vi "Polaris print label from powered unit.vi"(8 "error in (no error)":errorcluster, 10 "Baud":dbl=115200.0, 11 "VISA Refnum in":refnum<visa-resource-name>="COM11") -> (0 "error out":errorcluster)   [LabVIEW 2013]
panel:
  in  "Check label IMEI to unit?":bool
  out "IP":string
  out "Print Label OK?":bool=TRUE
  in  "Serial Number":u32
  in  "Printer name":string="\\\\LT-85LKFW2\\ZT230-300"
  out "ZPL final":string
  in  "ZPL template":string="\u0010CT~~CD,~CC^~CT~\n^XA~TA000~JSN^LT0^MNW^MTT^PON^PMN^LH0,0^JMA^PR4,4~SD28^JUS^LRN^CI0^XZ\n^FX Start of label zpl^FS\n^XA\n^MMT\n^PW750\n^LL0540\n^LS0\n^FT29,327^A0N,25,24^FH\\^FDNL PN: 1003071^FS\n^FT28,357^A0N,25,24^FH\\^FDIMEI: ImeiImeiImeiIme^FS\n^FT29,388^A0N,25,24^FH\\^FDICCID: EsimEsimEsimEsimEsim^FS\n^FT27,420^A0N,25,24^FH\\^FDSerial: WORKORDER^FS\n^FT28,451^A0N,22,22^FH\\^FDContains FCCID: RI7LE910CXWWX^FS\n^FT27,481^A0N,22,22^FH\\^FDContains IC: 5131A-LE910CXWWX^FS\n^FT359,327^A0N,21,21^FH\\^FDThis device complies with Part 15 of the^FS\n^FT359,353^A0N,21,21^FH\\^FDFCC Rules. Operation is subject to the^FS\n^FT359,379^A0N,21,21^FH\\^FDfollowing two conditions: (1) this device^FS\n^FT359,405^A0N,21,21^FH\\^FDmay not cause harmful interference, and^FS\n^FT359,431^A0N,21,21^FH\\^FD(2) this device must accept any interference^FS\n^FT359,457^A0N,21,21^FH\\^FDreceived, including interference that may^FS\n^FT359,483^A0N,21,21^FH\\^FDcause undesired operation.^FS\n^BY133,132^FT92,195^BXN,6,200,22,22,1,_\n^FH\\^FD4081093        EsimEsimEsimEsimEsim^FS\n^FT117,225^A0N,25,24^FH\\^FD4081093^FS\n^BY133,132^FT482,195^BXN,6,200,22,22,1,_\n^FH\\^FD3286910        ImeiImeiImeiIme^FS\n^FT500,228^A0N,25,24^FH\\^FD3286910^FS\n^FT459,256^A0N,25,24^FH\\^FDImeiImeiImeiIme^FS\n^FT59,253^A0N,25,24^FH\\^FDEsimEsimEsimEsimEsim^FS\n^PQ1,0,1,Y^XZ"
  out "imei":string
  out "eSim ICCID":string
  # "printer1=\\\\\\\\SkywireTestPC1\\ZDesigner ZT230-300dpi ZPL (Copy 1)\nprinter2=\\\\\\\\PucTestPC2\\ZDesigner ZT230-300dpi ZPL\nprinter3=\\\\\\\\NIMBELNKTESTPC3\\ZDesigner GX430t\nprinter4=\\\\\\\\dt-hkn77p2\\ZDesigner ZT230-200dpi ZPL\nprinter5=\\\\\\\\nimbelink-08\\ZDesigner ZT230-300dpi ZPL\nprinter6=\\\\\\\\LT-85LKFW2\\\\"
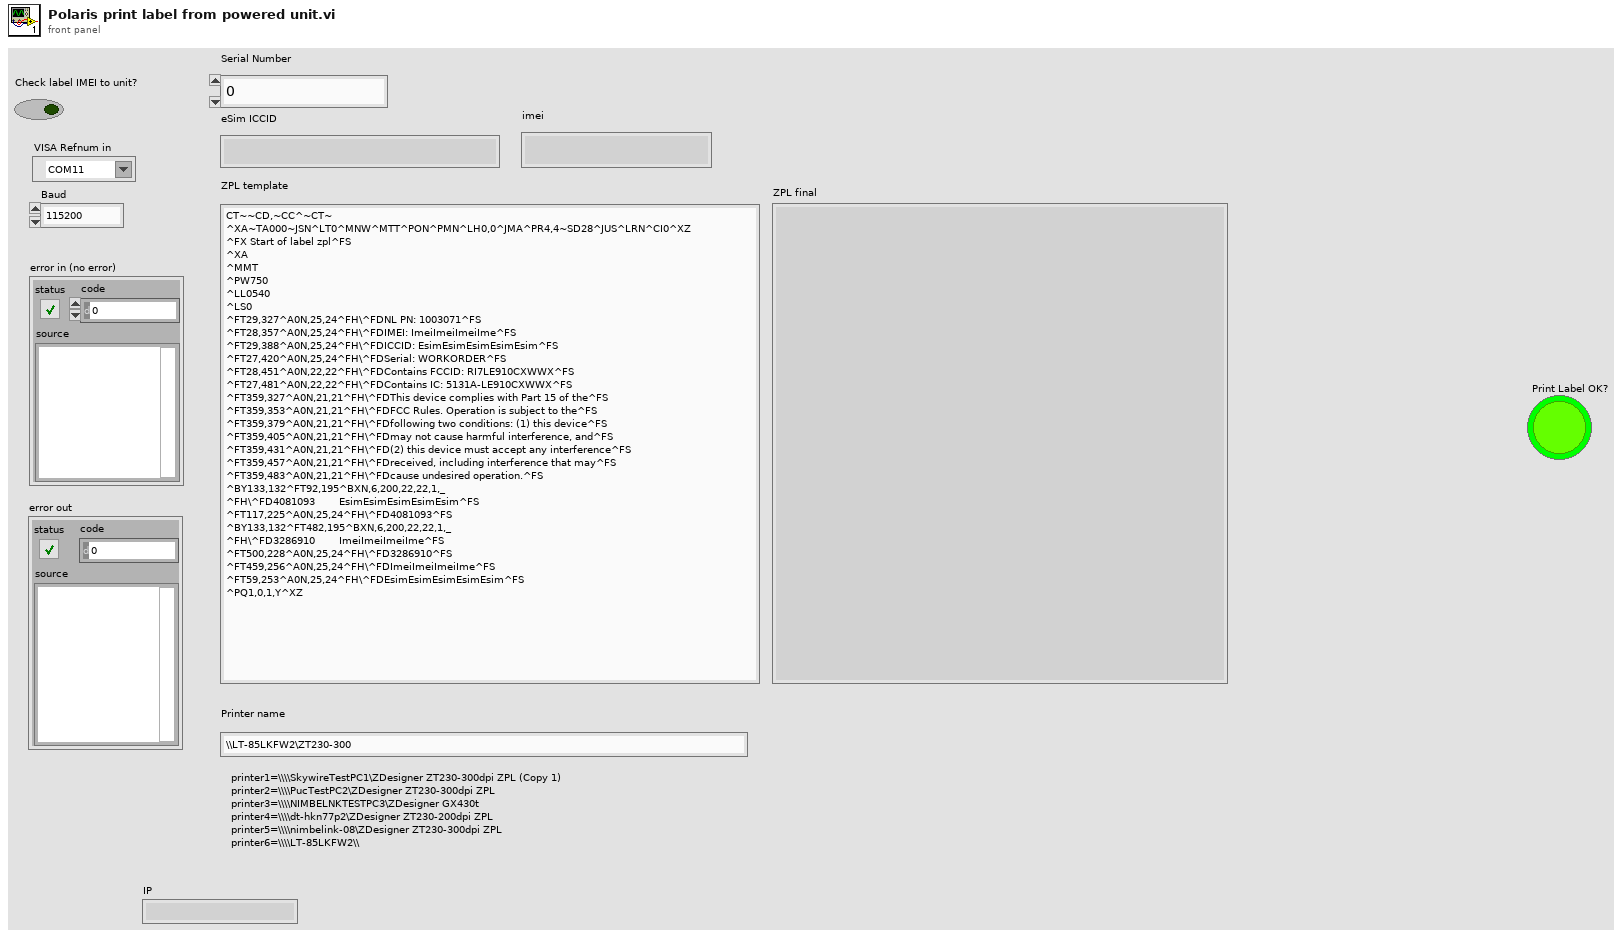
[diagram p1: front panel]
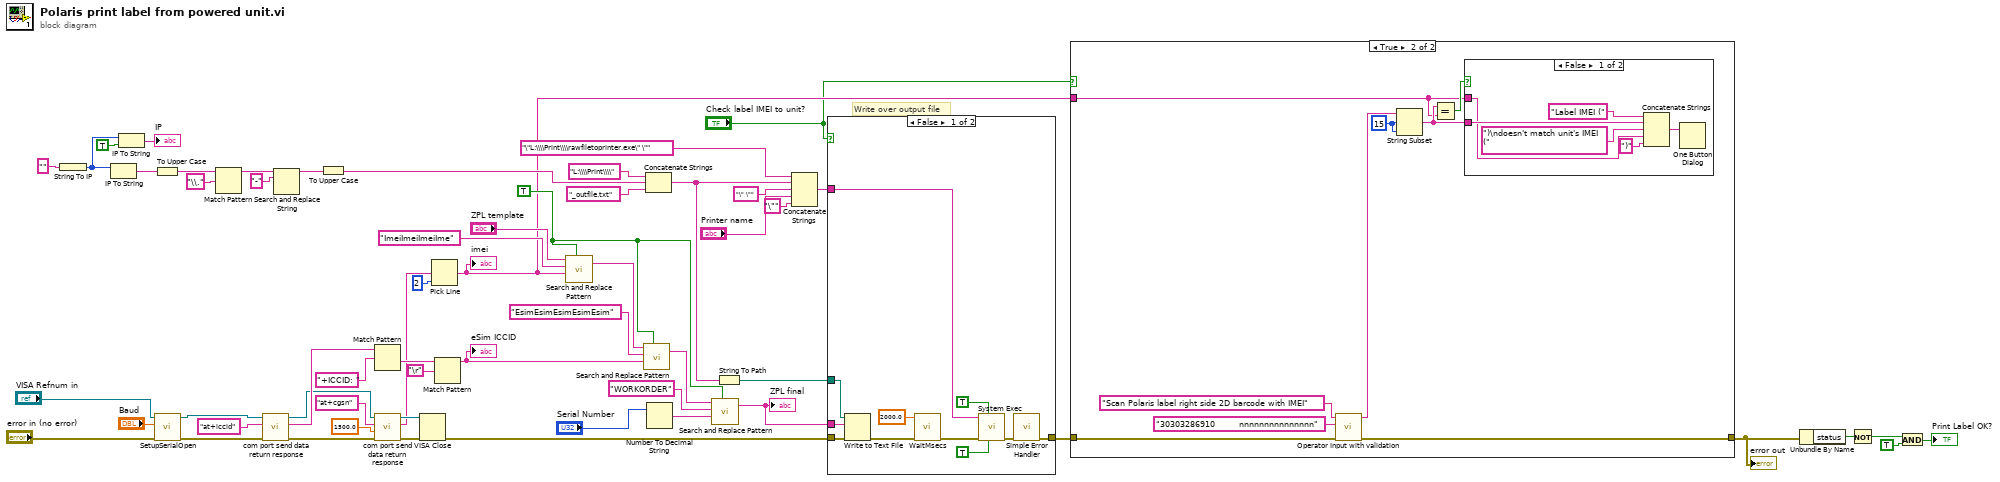
[diagram p0: block diagram]
diagram:
  w40 = TRUE ("replace all? (F)")
  # "Write over output file"
  n1 = String To IP(1:"" ("name")) -> (0:w23:u32)
  n2 = IP To String(2:w23) -> (0:w17:string)  [unwired: 1 in]
  n3 = IP To String(1:TRUE ("dot notation? (F)"), 2:w23) -> (0:→"IP":string)
  n4 = To Upper Case(1:w17) -> (0:w16:string)
  n5 = call "SetupSerialOpen.vi"("error in (no error)"="error in (no error)", "Baud"="Baud", "VISA Refnum in"="VISA Refnum in") -> ("error out"=w55:errorcluster, "VISA session"=w5:refnum<visa-resource-name>)  [unwired: 7 in]
  n6 = Match Pattern(string=w16, regular expression="\\.") -> (before substring=w20:string)  [unwired: 1 in, 3 out]
  n7 = call "com port send data return response.vi"("error in (no error)"=w55, "Send data"="at+iccid", "VISA resource name"=w5) -> ("error out"=w49:errorcluster, "response"=w51:string, "VISA resource name out"=w48:refnum<visa-resource-name>)  [unwired: 5 in, 1 out]
  n8 = Search and Replace String(input string=w20, search string="-") -> (result string=w18:string)  [unwired: 6 in, 3 out]
  n9 = To Upper Case(1:w18) -> (0:w15:string)
  n10 = Match Pattern(string=w51, regular expression="+ICCID: ") -> (after substring=w42:string)  [unwired: 1 in, 3 out]
  n11 = call "com port send data return response.vi"("error in (no error)"=w49, "Wait Msecs for response"=1500.0, "Send data"="at+cgsn", "VISA resource name"=w48) -> ("error out"=w36:errorcluster, "response"=w9:string, "VISA resource name out"=w47:refnum<visa-resource-name>)  [unwired: 4 in, 1 out]
  n12 = VISA Close(VISA resource name=w47, error in (no error)=w36) -> (error out=w12:errorcluster)
  n13 = Pick Line(multi-line string=w9, line index=2) -> (output string=w4:string)  [unwired: 1 in]
  "imei" <- w4
  n14 = Match Pattern(string=w42, regular expression="\r") -> (before substring=w6:string)  [unwired: 1 in, 3 out]
  "eSim ICCID" <- w6
  n15 = call <vilib>:"Search and Replace Pattern.vi"("string"="ZPL template", "regular expression (\"\")"="ImeiImeiImeiIme" ("string"), "replace string (\"\")"=w4, "replace all? (F)"=w40) -> ("result string"=w44:string)  [unwired: 1 in, 1 out]
  n16 = call <vilib>:"Search and Replace Pattern.vi"("string"=w44, "regular expression (\"\")"="EsimEsimEsimEsimEsim" ("regular expression (\"\")"), "replace string (\"\")"=w6, "replace all? (F)"=w40) -> ("result string"=w41:string)  [unwired: 1 in, 1 out]
  n17 = Concatenate Strings("L:\\\\Print\\\\" ("string"), w15, "_outfile.txt" ("string")) -> (w26:string)
  n18 = Number To Decimal String(number="Serial Number") -> (decimal integer string=w37:string)  [unwired: 1 in]
  n19 = call <vilib>:"Search and Replace Pattern.vi"("string"=w41, "regular expression (\"\")"="WORKORDER" ("regular expression (\"\")"), "replace string (\"\")"=w37, "replace all? (F)"=w40) -> ("result string"=w11:string)  [unwired: 1 in, 1 out]
  "ZPL final" <- w11
  n20 = String To Path(string=w26) -> (path=w14:path)
  n21 = Concatenate Strings("\"L:\\\\Print\\\\rawfiletoprinter.exe\" \"" ("string"), w26, "\" \"" ("string"), "Printer name", "\"" ("string")) -> (w13:string)
  n22 = case shown="False" "Check label IMEI to unit?" {
    tunnel: w14 -> [w64 _]
    tunnel: w13 -> [w62 _]
    tunnel: w12 -> [w61 w70]
    tunnel: w11 -> [w60 _]
    tunnel: [w59 w70] -> w2
    frame False {
      n23 = Write to Text File(file (use dialog)=w64, text=w60, error in=w61) -> (error out=w63:errorcluster)  [unwired: 1 in, 2 out]
      n24 = call "WaitMsecs.vi"("error in (no error)"=w63, "Wait Msecs"=2000.0) -> ("error out"=w66:errorcluster)  [unwired: 9 in]
      n25 = call <vilib>:"System Exec.vi"("run minimized? (F)"=TRUE, "wait until completion? (T)"=TRUE, "error in (no error)"=w66, "command line"=w62) -> ("error out"=w67:errorcluster)  [unwired: 4 in, 3 out]
      n26 = call <vilib>:"Simple Error Handler.vi"("error in (no error)"=w67) -> ("error out"=w59:errorcluster)  [unwired: 4 in, 4 out]
    }
    frame True {
    }
  }
  n27 = case shown="True" "Check label IMEI to unit?" {
    tunnel: w4 -> [_ w72]
    tunnel: w2 -> [w71 w76]
    tunnel: [w71 w75] -> w1
    frame False {
    }
    frame True {
      w78 = 15 ("offset (0)")
      n28 = call "Operator Input with validation.vi"("error in (no error)"=w76, "Validation string"="30303286910        nnnnnnnnnnnnnnn", "Message"="Scan Polaris label right side 2D barcode with IMEI") -> ("error out"=w75:errorcluster, "Response"=w79:string)  [unwired: 6 in, 1 out]
      n29 = String Subset(string=w79, offset (0)=w78, length (rest)=w78) -> (substring=w73:string)
      n30 = Equal?(x=w73, y=w72) -> (x = y?=w74:bool)
      n31 = case shown="False" w74 {
        tunnel: w73 -> [w85 _]
        tunnel: w72 -> [w83 _]
        frame False {
          n32 = Concatenate Strings("Label IMEI (" ("string"), w85, ")\ndoesn't match unit's IMEI (" ("string"), w83, ")" ("string")) -> (w81:string)
          n33 = One Button Dialog(message=w81) -> ()  [unwired: 1 in, 1 out]
        }
        frame True {
        }
      }
    }
  }
  "error out" <- w1
  n34 = Unbundle By Name(w1) -> ("status"=w33:bool)
  n35 = Not(x=w33) -> (.not. x?=w32:bool)
  n36 = And(x=w32, y=TRUE) -> (x .and. y?=→"Print Label OK?":bool)
